vi "Write Weight Type.vi"(8 "error in":errorcluster, 10 "Weight Type":T1, 11 "GrabberTool in":refnum<class "GrabberTool Class.lvclass">) -> (0 "error out":errorcluster, 3 "GrabberTool out":refnum<class "GrabberTool Class.lvclass">)   [LabVIEW 2011, in "GrabberTool Class.lvclass"]
uses:
  GrabberTool Class.lvclass
  Config Manager Class/Type Definitions/Weight Type.ctl
  GrabberTool Class.lvclass/GrabberTool Class.ctl
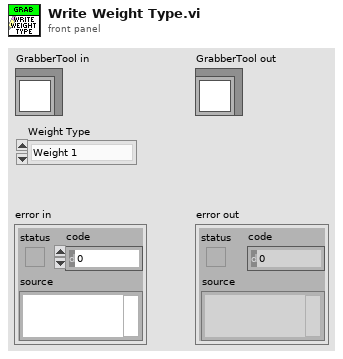
[diagram p1: front panel]
types:
  T1 = typedef "Weight Type.ctl" = enum16{"Weight 1", "Weight 2", "Weight 3", "Weight 4", "Weight 5", "Weight 6", "Weight 7", "Weight 8"}
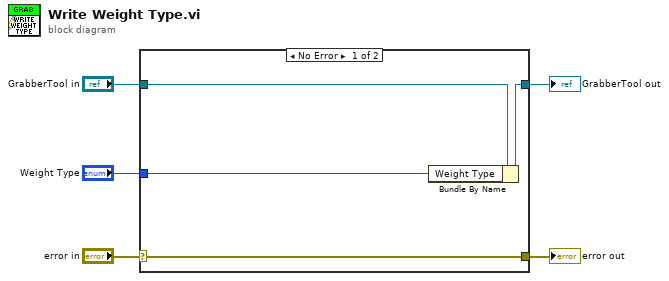
[diagram p0: block diagram]
diagram:
  n1 = case shown="No Error" "error in" {
    selector: "error in" -> [w9 w10]
    tunnel: [w9 w10] -> w4
    tunnel: [w7 w11] -> w2
    tunnel: "GrabberTool in" -> [w8 w11]
    tunnel: "Weight Type" -> [w6 _]
    frame No Error {
      n2 = Bundle By Name(cluster=w8, "Weight Type"=w6) -> (w7:refnum<class "GrabberTool Class.lvclass">)
    }
    frame Error {
    }
  }
  "error out" <- w4
  "GrabberTool out" <- w2
